vi "EncoderBegin.vi"() -> ()   [LabVIEW 2013]
uses:
  <vilib>/Rock Robotics/SystemInterfaces/DIO/FPGA_DIOChannel.ctl
  <vilib>/Rock Robotics/SystemInterfaces/Typedef/FPGA_TypedefDigitalModule.ctl
  <vilib>/Rock Robotics/WPI/Encoder/WPI_EncoderType.ctl
  <vilib>/Rock Robotics/WPI/Counter/WPI_CounterDigitalInputToDigitalSource.vi
panel:
  out "error out":errorcluster
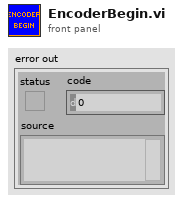
[diagram p1: front panel]
types:
  T1 = typedef "WPI_EncoderType.ctl" = enum16{"1x", "2x", "4x"}
  T2 = typedef "FPGA_TypedefDigitalModule.ctl" = enum16{"Digital Module 1", "Digital Module 2"}
  T3 = typedef "FPGA_DIOChannel.ctl" = enum8{"DIO 1", "DIO 2", "DIO 3", "DIO 4", "DIO 5", "DIO 6", "DIO 7", "DIO 8", "DIO 9", "DIO 10", "DIO 11", "DIO 12", "DIO 13", "DIO 14", "Invalid"}
  T4 = typedef "WPI_DigitalInputDevRef.ctl" = cluster{"DevStatus":errorcluster, "DIO Channel":T3, "Digital Module":T2}
  T5 = typedef "FPGA_CounterEncoderSourceConvertionLVSourceType.ctl" = cluster{"DevStatus":errorcluster, "AnalogTriggerMode?":bool, "DigitalMode":cluster{"Digital Module":T2, "DIO Channel":T6}, "AnalogTriggerMode":cluster{"AnalogTriggerIndex":T7, "OutputType":T8}}
  T6 = typedef "FPGA_DIODigitalSourceChannel.ctl" = enum8{"DIO 1", "DIO 2", "DIO 3", "DIO 4", "DIO 5", "DIO 6", "DIO 7", "DIO 8", "DIO 9", "DIO 10", "DIO 11", "DIO 12", "DIO 13", "DIO 14", "Disabled"}
  T7 = typedef "FPGA_AnalogTriggerIndex.ctl" = enum8{"Trig 0", "Trig 1", "Trig 2", "Trig 3", "Trig 4", "Trig 5", "Trig 6", "Trig 7", "Invalid"}
  T8 = typedef "FPGA_AnalogTriggerOutType.ctl" = enum16{"InWindow", "TriggerState", "Rising", "Falling"}
  T9 = typedef "WPI_EncoderDevRef.ctl" = cluster{"DevStatus":errorcluster, "EncoderIndex":T10, "CounterIndex":T11, "DistancePerCount":dbl, "Decoding Type":T1}
  T10 = typedef "FPGA_EncoderIdx.ctl" = enum8{"Enc 0", "Enc 1", "Enc 2", "Enc 3", "Invalid"}
  T11 = typedef "FPGA_CounterCtrSystemIndex.ctl" = enum8{"Ctr 0", "Ctr 1", "Ctr 2", "Ctr 3", "Ctr 4", "Ctr 5", "Ctr 6", "Ctr 7", "Invalid"}
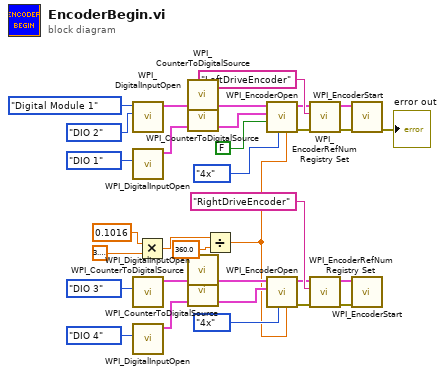
[diagram p0: block diagram]
diagram:
  n1 = call <vilib>:"WPI_DigitalInputOpen.vi"("DIO Channel"=FPGA_DIOChannel."DIO 2", "Digital Module (Module 1)"=FPGA_TypedefDigitalModule."Digital Module 1") -> ("DigitalInputDevRef"=w16:T4)  [unwired: 8 in, 1 out]
  n2 = call <vilib>:"WPI_DigitalInputOpen.vi"("DIO Channel"=FPGA_DIOChannel."DIO 1") -> ("DigitalInputDevRef"=w18:T4)  [unwired: 9 in, 1 out]
  n3 = call <vilib>:"WPI_DigitalInputOpen.vi"("DIO Channel"=FPGA_DIOChannel."DIO 3") -> ("DigitalInputDevRef"=w25:T4)  [unwired: 9 in, 1 out]
  n4 = call <vilib>:"WPI_DigitalInputOpen.vi"("DIO Channel"=FPGA_DIOChannel."DIO 4") -> ("DigitalInputDevRef"=w27:T4)  [unwired: 9 in, 1 out]
  n5 = Multiply(x=0.1016, y=3.141592653589793) -> (x*y=w2:dbl)
  n6 = call-poly <vilib>:"WPI_CounterToDigitalSource.vi"("DigitalInputDevRef"=w16) -> ("Digital Source"=w19:T5)  [unwired: 6 in]
  n7 = call-poly <vilib>:"WPI_CounterToDigitalSource.vi"("DigitalInputDevRef"=w18) -> ("Digital Source"=w20:T5)  [unwired: 6 in]
  n8 = call-poly <vilib>:"WPI_CounterToDigitalSource.vi"("DigitalInputDevRef"=w25) -> ("Digital Source"=w28:T5)  [unwired: 6 in]
  n9 = call-poly <vilib>:"WPI_CounterToDigitalSource.vi"("DigitalInputDevRef"=w27) -> ("Digital Source"=w29:T5)  [unwired: 6 in]
  n10 = Divide(x=w2, y=360.0) -> (x/y=w1:dbl)
  n11 = call <vilib>:"WPI_EncoderOpen.vi"("DistancePerCount"=w1, "Decoding Type"=WPI_EncoderType."4x", "Invert Direction (False)"=FALSE, "BSource"=w20, "ASource"=w19) -> ("error out"=w21:errorcluster, "EncoderDevRef"=w22:T9)  [unwired: 5 in]
  n12 = call <vilib>:"WPI_EncoderOpen.vi"("DistancePerCount"=w1, "Decoding Type"=WPI_EncoderType."4x", "BSource"=w29, "ASource"=w28) -> ("error out"=w30:errorcluster, "EncoderDevRef"=w31:T9)  [unwired: 6 in]
  n13 = call <vilib>:"WPI_EncoderRefNum Registry Set.vi"("error in (no error)"=w21, "refnum name"="LeftDriveEncoder", "EncoderDevRef"=w22) -> ("error out"=w12:errorcluster, "EncoderDevRef"=w13:T9)  [unwired: 7 in]
  n14 = call <vilib>:"WPI_EncoderRefNum Registry Set.vi"("error in (no error)"=w30, "refnum name"="RightDriveEncoder", "EncoderDevRef"=w31) -> ("error out"=w9:errorcluster, "EncoderDevRef"=w10:T9)  [unwired: 7 in]
  n15 = call <vilib>:"WPI_EncoderStart.vi"("error in (no error)"=w12, "EncoderDevRef"=w13) -> ("error out"=→"error out":errorcluster)  [unwired: 8 in, 1 out]
  n16 = call <vilib>:"WPI_EncoderStart.vi"("error in (no error)"=w9, "EncoderDevRef"=w10) -> ()  [unwired: 8 in, 2 out]
